vi "Fill Colors.vi"(6 "Dim":u8=1 min=1 step=1, 8 "error in (no error)":errorcluster, 9 "Cluster":T1, 11 "Refnum in":refnum<k20>) -> (0 "error out":errorcluster, 3 "Refnum out":refnum<k20>, 5 "LED Matrix":picture)   [LabVIEW 2013]
uses:
  Cluser.ctl
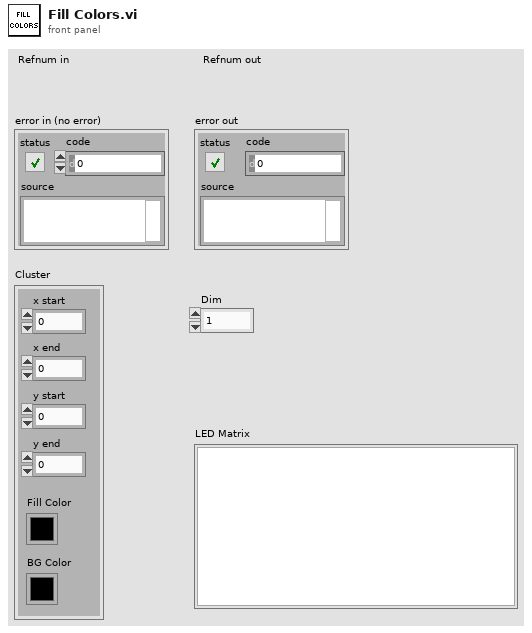
[diagram p1: front panel]
types:
  T1 = typedef "Cluser.ctl" = cluster{"x start":u16, "x end":u16, "y start":u16, "y end":u16, "Fill Color":u32, "BG Color":u32}
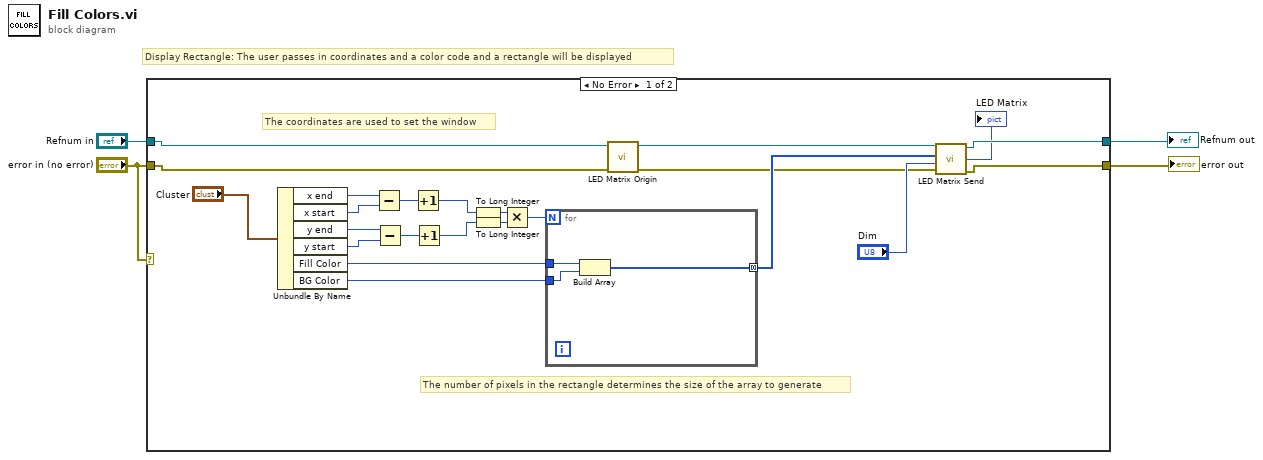
[diagram p0: block diagram]
diagram:
  # "Display Rectangle: The user passes in coordinates and a color code and a rectangle will be displayed"
  n1 = case shown="No Error" "error in (no error)" {
    tunnel: "error in (no error)" -> [w8 w31]
    tunnel: "Refnum in" -> [w9 w32]
    tunnel: [w13 w32] -> w1
    tunnel: [w12 w31] -> w3
    frame No Error {
      # "The number of pixels in the rectangle determines the size of the array to generate"
      # "The coordinates are used to set the window"
      n2 = Unbundle By Name("Cluster") -> ("x end"=w26:u16, "x start"=w25:u16, "y end"=w24:u16, "y start"=w23:u16, "Fill Color"=w18:u32, "BG Color"=w17:u32)
      n3 = Subtract(x=w26, y=w25) -> (x-y=w22:u16)
      n4 = Subtract(x=w24, y=w23) -> (x-y=w21:u16)
      n5 = Increment(x=w22) -> (x+1=w16:u16)
      n6 = Increment(x=w21) -> (x+1=w15:u16)
      n7 = To Long Integer(number=w16) -> (32bit integer=w20:i32)
      n8 = To Long Integer(number=w15) -> (32bit integer=w19:i32)
      n9 = Multiply(x=w20, y=w19) -> (x*y=w14:i32)
      n10 = for {
        N: w14 -> [_]
        tunnel: w18 -> [w30]
        tunnel: w17 -> [w29]
        tunnel: [w28] -> w11 mode=concatenating
        n11 = Build Array(w30, w29) -> (w28:u32[])
      }
      n12 = call "LED Matrix Origin.vi"("error in (no error)"=w8, "Refnum in"=w9) -> ("error out"=w7:errorcluster, "Refnum out"=w6:refnum<k20>)  [unwired: 8 in]
      n13 = call "LED Matrix Send.vi"("error in (no error)"=w7, "Brightness"="Dim", "Data"=w11, "Refnum in"=w6) -> ("error out"=w12:errorcluster, "Refnum out"=w13:refnum<k20>, "LED Matrix"=→"LED Matrix":picture)  [unwired: 4 in]
    }
    frame Error {
    }
  }
  "error out" <- w3
  "Refnum out" <- w1
